vi "ErrorHandling.ClearErrorHistory.vi"(8 "error IO":errorcluster) -> (0 "error IO":errorcluster)   [LabVIEW 2016, in "ErrorHandling.lvclass"]
uses:
  ErrorHandling.lvclass
  ErrorHandling.lvclass/ErrorHandling.ctl
  ErrorHandling.OccurredErrorDataStruct.ctl
  Package Libraries/Message Queue/MessageQueue_GetQueue.vi
  Package Libraries/Message Queue/MessageQueue_EnqueueElement.vi
  Package Libraries/Message Queue/MessageQueue_DequeueElement.vi
  Package Libraries/Message Queue/MessageQueue_ReleaseQueue.vi
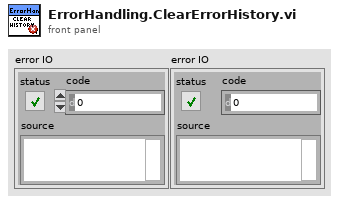
[diagram p1: front panel]
types:
  T1 = typedef "ErrorHandling.lvclass/ErrorHandling.OccurredErrorDataStruct.ctl" = cluster{"Error":errorcluster, "Caller":string, "Comment":string, "Timestamp":timestamp, "Stopped":bool, "ErrorCusterString":string, "ErrorIndex":u64}
  T2 = enum16{"open", "replace", "create", "open or create", "replace or create", "replace or create with confirmation"}
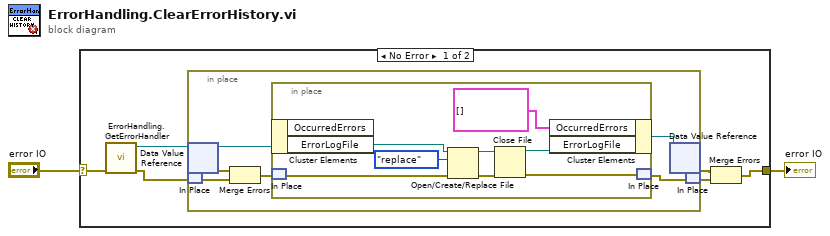
[diagram p0: block diagram]
diagram:
  n1 = case shown="No Error" "error IO" {
    selector: "error IO" -> [w8 w23]
    tunnel: [w5 w23] -> w1
    frame No Error {
      n2 = call "ErrorHandling.GetErrorHandler.vi"("ErrorIn"=w8) -> ("ErrorOut"=w6:errorcluster, "ErrorRef"=w7:refnum<data-value>)  [unwired: 8 in, 1 out]
      n3 = in-place {
        n4 = in-place-dvr #1(w7) -> (w12:refnum<class "ErrorHandling.lvclass">, w14:errorcluster)
        n5 = in-place-match #2(w6) -> (w13:errorcluster)
        n6 = Merge Errors(w14, w13) -> (w11:errorcluster)
        n7 = in-place {
          n8 = in-place-cluster #3(w12) -> ("ErrorLogFile"=w22:path)  [unwired: 1 out]
          n9 = in-place-match #4(w11) -> (w17:errorcluster)
          n10 = Open/Create/Replace File(file path (use dialog)=w22, error in=w17, operation (0:open)=T2."replace") -> (refnum out=w19:refnum<file>, error out=w20:errorcluster)  [unwired: 3 in, 1 out]
          n11 = Close File(refnum=w19, error in=w20) -> (path=w18:path, error out=w16:errorcluster)
          n12 = in-place-cluster #3("OccurredErrors"=T1[] [], "ErrorLogFile"=w18) -> (w9:refnum<class "ErrorHandling.lvclass">)
          n13 = in-place-match #4(w16) -> (w10:errorcluster)
        }
        n14 = in-place-dvr #1(w9) -> (w3:errorcluster)  [unwired: 1 out]
        n15 = in-place-match #2(w10) -> (w4:errorcluster)
      }
      n16 = Merge Errors(w3, w4) -> (w5:errorcluster)
    }
    frame Error {
    }
  }
  "error IO" <- w1
